vi "Przełącznik R-S.vi"(8 "S":bool, 11 "R":bool) -> (0 "~Q":bool, 3 "Q":bool)   [LabVIEW 2020]
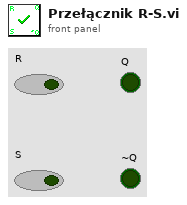
[diagram p1: front panel]
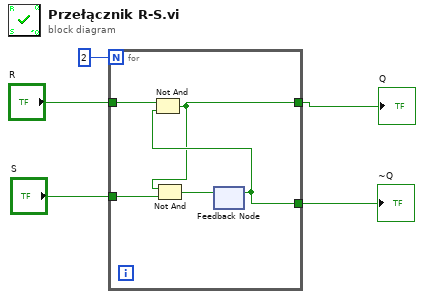
[diagram p0: block diagram]
diagram:
  n1 = for {
    N: 2 -> [_]
    tunnel: "S" -> [w9]
    tunnel: [w7] -> w4
    tunnel: "R" -> [w10]
    tunnel: [w6] -> w5
    n2 = feedback #1() -> (w7:bool)  [unwired: 1 in]
    n3 = Not And(1:w7, 2:w10) -> (0:w6:bool)
    n4 = Not And(1:w9, 2:w6) -> (0:w8:bool)
    n5 = feedback-in #1(w8) -> ()
  }
  "Q" <- w5
  "~Q" <- w4
